vi "UpdateAddDeviceMenu.vi"(8 "error in":errorcluster, 11 "AddDeviceMenu in":refnum<vi>) -> (0 "error out":errorcluster, 3 "AddDeviceMenu out":refnum<vi>)   [LabVIEW 2013]
uses:
  TypeDefs/AddDeviceRing.ctl
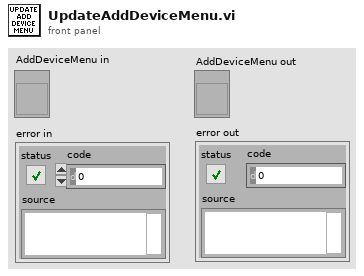
[diagram p1: front panel]
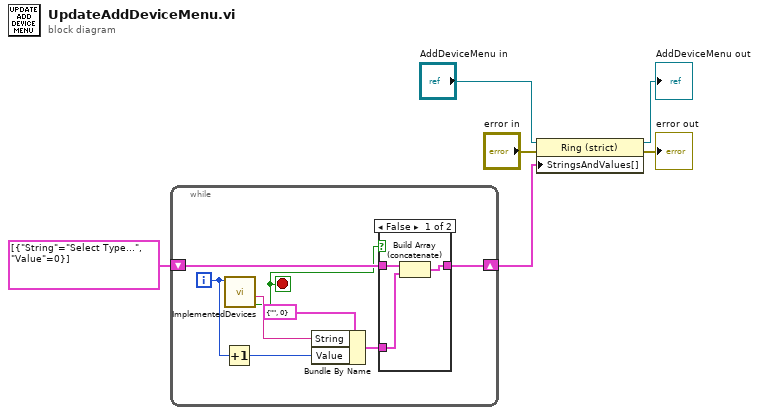
[diagram p0: block diagram]
diagram:
  n1 = while {
    shift-right: [w12] -> w4
    shift-left: cluster{"String":string, "Value":u16}[] [{"String"="Select Type...", "Value"=0}] -> [w11]
    i -> [w9]
    stop <- w7 stop-if-true
    n2 = Increment(x=w9) -> (x+1=w8:i32)
    n3 = call "ImplementedDevices.vi"("Index"=w9) -> ("Not In List"=w7:bool, "Menu Name"=w10:string)  [unwired: 8 in, 1 out]
    n4 = Bundle By Name(cluster=cluster{"String":string, "Value":u16} {"String"="", "Value"=0}, "String"=w10, "Value"=w8) -> (w13:cluster{"String":string, "Value":u16})
    n5 = case shown="False" w7 {
      tunnel: w13 -> [w17 _]
      tunnel: [w16 w18] -> w12
      tunnel: w11 -> [w15 w18]
      frame False {
        n6 = Build Array (concatenate)(w15, w17) -> (w16:cluster{"String":string, "Value":u16}[])
      }
      frame True {
      }
    }
  }
  n7 = property class="Ring (strict)"(reference="AddDeviceMenu in", error in="error in", "StringsAndValues[]"=w4) -> (reference out=→"AddDeviceMenu out":refnum<vi>, error out=→"error out":errorcluster)
